vi "fan moving.vi"() -> ()   [LabVIEW 2020]
panel:
  in  "speed":dbl(knob) scale=0.0..10.0
  in  "stop":bool
  out "fan":u16(ring)
  # "high"
  # "low"
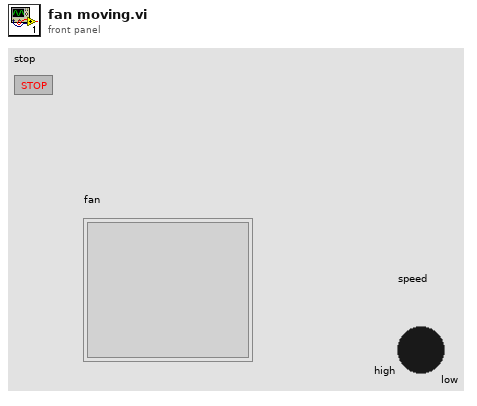
[diagram p1: front panel]
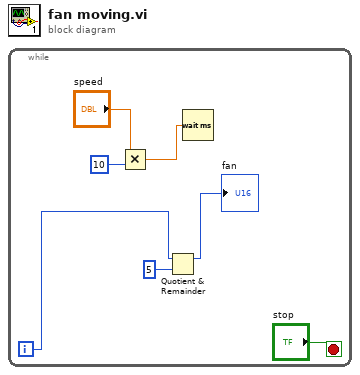
[diagram p0: block diagram]
diagram:
  n1 = while {
    i -> [w4]
    stop <- "stop" stop-if-true
    n2 = Multiply(x="speed", y=10) -> (x*y=w5:dbl)
    n3 = Quotient & Remainder(x=w4, y=5) -> (x-y*floor(x/y)=→"fan":i32)  [unwired: 1 out]
    n4 = Wait (ms)(milliseconds to wait=w5) -> ()  [unwired: 1 out]
  }
